vi "Define Alarms.vi"(8 "error in (no error)":errorcluster, 11 "SE_SECSGEM in":refnum<class "SE_SECSGEM.lvclass">=refnum) -> (0 "error out":errorcluster, 3 "SE_SECSGEM out":refnum<class "SE_SECSGEM.lvclass">)   [LabVIEW 2022 SP3, in "SE_SECSGEM.lvclass"]
uses:
  SE_SECSGEM.lvclass
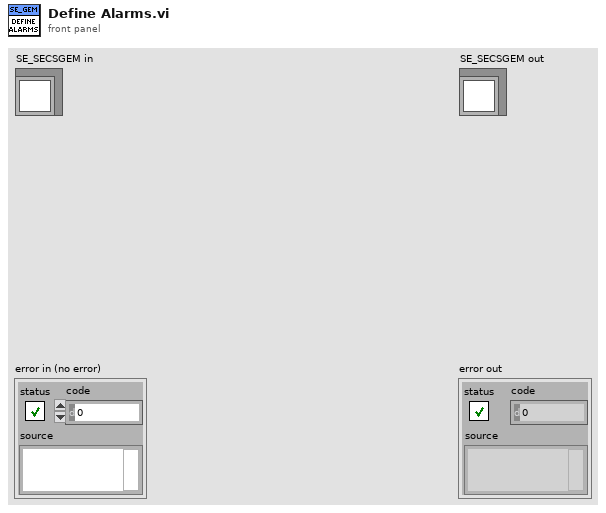
[diagram p1: front panel]
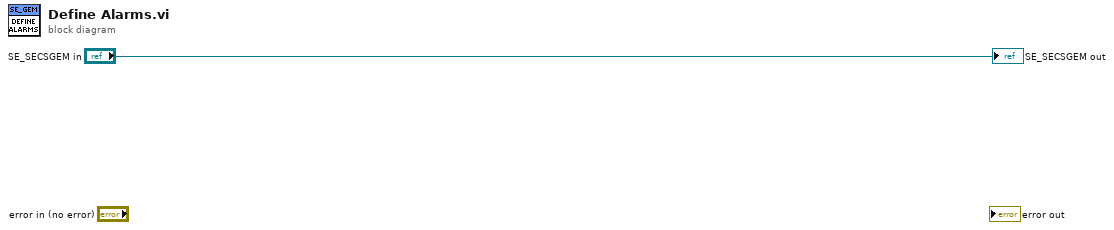
[diagram p0: block diagram]
diagram:
  "SE_SECSGEM out" <- "SE_SECSGEM in"
